vi "Toggle Stream.vi"(8 "error in (no error)":errorcluster, 11 "OBS in":refnum<class "OBS.lvclass">) -> (0 "error out":errorcluster, 2 "Active":bool, 3 "OBS out":refnum<class "OBS.lvclass">)   [LabVIEW 2020, in "obs-websocket.lvlib" / "OBS.lvclass"]
uses:
  OBS.lvclass
  OBS.lvclass/OBS.ctl
  ToggleStream/ToggleStream.lvclass
  RToggleStream/RToggleStream.lvclass
  C:/dev/lv20CE/lv-obs-websocket/obs-websocket-lv/Response/Response.lvclass
  C:/dev/lv20CE/lv-obs-websocket/obs-websocket-lv/Server Message/Server Message.lvclass
  C:/dev/lv20CE/lv-obs-websocket/obs-websocket-lv/Message/Message.lvclass
  C:/dev/lv20CE/lv-obs-websocket/obs-websocket-lv/RToggleStream/RToggleStream.lvclass
  C:/dev/lv20CE/lv-obs-websocket/obs-websocket-lv/Request/Request.lvclass
  C:/dev/lv20CE/lv-obs-websocket/obs-websocket-lv/Client Message/Client Message.lvclass
  C:/dev/lv20CE/lv-obs-websocket/obs-websocket-lv/ToggleStream/ToggleStream.lvclass
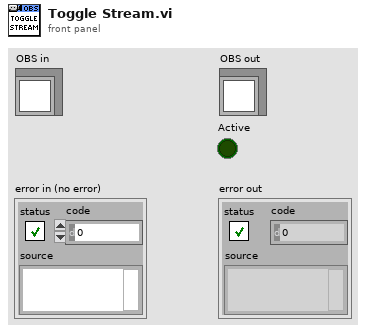
[diagram p1: front panel]
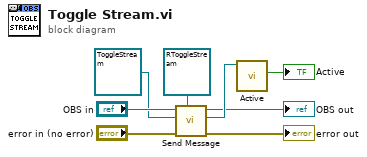
[diagram p0: block diagram]
diagram:
  n1 = call "Send Message.vi"("Response Type (None)"=refnum<class "RToggleStream.lvclass"> refnum ("obs-websocket-lv.lvlib:RToggleStream.lvclass"), "error in (no error)"="error in (no error)", "Client Message"=refnum<class "ToggleStream.lvclass"> refnum ("obs-websocket-lv.lvlib:ToggleStream.lvclass"), "OBS in"="OBS in") -> ("error out"=→"error out":errorcluster, "Response"=w4:refnum<class "RToggleStream.lvclass">, "OBS out"=→"OBS out":refnum<class "OBS.lvclass">)  [unwired: 4 in, 1 out]
  n2 = call "Active.vi"("RToggleStream in"=w4) -> ("Active"=→"Active":bool)  [unwired: 8 in, 2 out]
